vi "Update VI Description.vi"   [LabVIEW 2015]
doc: "<b> </b> <b> </b>\n©2016 Q Software Innovations, LLC (QSI)\nwritten by Quentin Alldredge\nproduced in LabVIEW 2015"
uses:
  Project Manipulation Scripts/Project Manipulation Scripts.lvlib
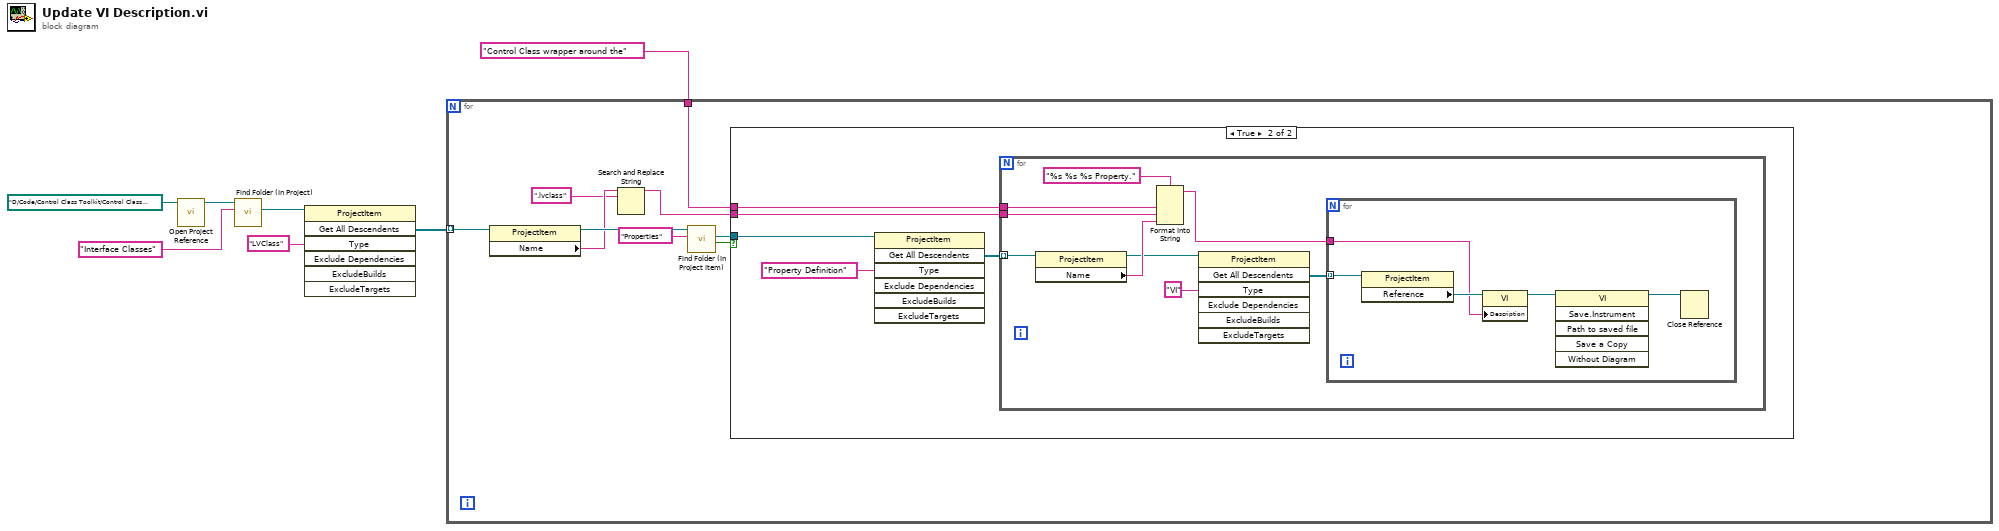
[diagram p0: block diagram]
diagram:
  n1 = call "Open Project Reference.vi"("Project Path"=path "D:/Code/Control Class Toolkit/Control Class Toolkit.lvproj") -> ("Project out"=w6:refnum<vi>)  [unwired: 10 in]
  n2 = call "Find Folder (In Project).vi"("Folder Name"="Interface Classes", "Project in"=w6) -> ("Folder Refnum"=w4:refnum<vi>)  [unwired: 7 in, 2 out]
  n3 = invoke class="ProjectItem" method="Get All Descendents"(reference=w4, "Type"="LVClass") -> ("All Descendents"=w2:refnum<vi>[])  [unwired: 5 in, 6 out]
  n4 = for {
    tunnel: w2 -> [w13] mode=indexing
    tunnel: "Control Class wrapper around the" ("Folder Name") -> [w11]
    n5 = property class="ProjectItem"(reference=w13) -> (reference out=w12:refnum<vi>, "Name"=w10:string)  [unwired: 1 in, 1 out]
    n6 = Search and Replace String(input string=w10, search string=".lvclass" ("format string")) -> (result string=w8:string)  [unwired: 6 in, 3 out]
    n7 = call "Find Folder (In Project Item).vi"("Folder Name"="Properties", "ProjectItem in"=w12) -> ("Found?"=w14:bool, "Folder Refnum"=w15:refnum<vi>)  [unwired: 7 in, 1 out]
    n8 = case shown="True" w14 {
      tunnel: w15 -> [_ w21]
      tunnel: w8 -> [_ w18]
      tunnel: w11 -> [_ w17]
      frame False {
      }
      frame True {
        n9 = invoke class="ProjectItem" method="Get All Descendents"(reference=w21, "Type"="Property Definition") -> ("All Descendents"=w20:refnum<vi>[])  [unwired: 5 in, 6 out]
        n10 = for {
          tunnel: w20 -> [w30] mode=indexing
          tunnel: w18 -> [w27]
          tunnel: w17 -> [w28]
          n11 = property class="ProjectItem"(reference=w30) -> (reference out=w24:refnum<vi>, "Name"=w26:string)  [unwired: 1 in, 1 out]
          n12 = Format Into String(format string="%s %s %s Property.", w28, w27, w26) -> (resulting string=w22:string)  [unwired: 2 in, 1 out]
          n13 = invoke class="ProjectItem" method="Get All Descendents"(reference=w24, "Type"="VI") -> ("All Descendents"=w23:refnum<vi>[])  [unwired: 5 in, 6 out]
          n14 = for {
            tunnel: w23 -> [w35] mode=indexing
            tunnel: w22 -> [w33]
            n15 = property class="ProjectItem"(reference=w35) -> ("Reference"=w34:refnum<vi>)  [unwired: 1 in, 2 out]
            n16 = property class="VI"(reference=w34, "Description"=w33) -> (reference out=w32:refnum<vi>)  [unwired: 1 in, 1 out]
            n17 = invoke class="VI" method="Save.Instrument"(reference=w32) -> (reference out=w31:refnum<vi>)  [unwired: 5 in, 5 out]
            n18 = Close Reference(reference=w31) -> ()  [unwired: 1 in, 1 out]
          }
        }
      }
    }
  }
